vi "ExcelWrite.vi"(6 "Start Position":cluster{"Sheet":i32, "Row":i32, "Column":i32}={"Sheet"=0, "Row"=1, "Column"=2}, 9 "Values":string[][][](array[string]), 10 "Report Name":path, 11 "Module File":path) -> ()   [LabVIEW 2014]
uses:
  Data/Polymorphic VIs/Set Cell (String).vi
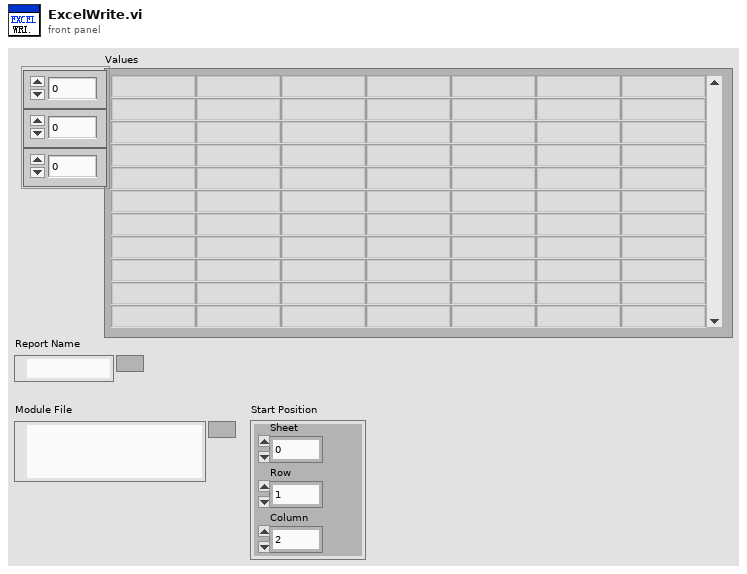
[diagram p1: front panel]
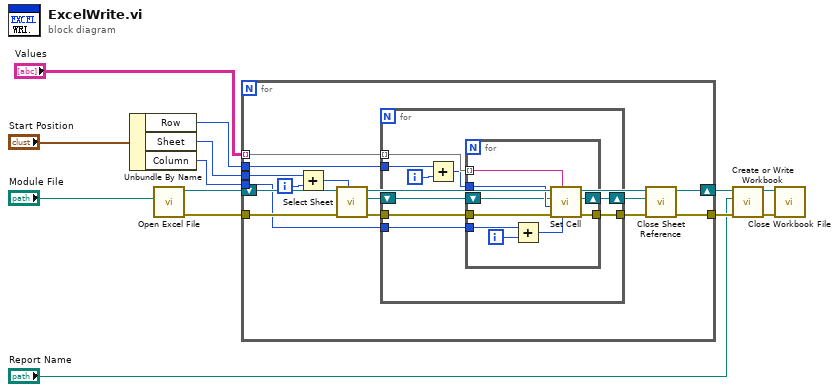
[diagram p0: block diagram]
diagram:
  n1 = Unbundle By Name("Start Position") -> ("Row"=w11:i32, "Sheet"=w5:i32, "Column"=w4:i32)
  n2 = call "Open Excel File.vi"("File Name"="Module File") -> ("error out"=w10:errorcluster, "IWorkbook Reference Out"=w13:refnum<k24>)  [unwired: 9 in]
  n3 = for {
    tunnel: "Values" -> [w21] mode=indexing
    tunnel: w5 -> [w25]
    tunnel: w4 -> [w19]
    tunnel: w11 -> [w20]
    tunnel: w10 -> [w23]
    tunnel: [w15] -> w9
    shift-right: [w22] -> w8
    shift-left: w13 -> [w27]
    i -> [w26]
    n4 = Add(x=w25, y=w26) -> (x+y=w24:i32)
    n5 = call "Select Sheet.vi"("Sheet (0)"=w24, "error in (no error)"=w23, "IWorkbook Reference"=w27) -> ("error out"=w18:errorcluster, "Sheet Reference"=w14:refnum<k24>, "IWorkbook Reference"=w22:refnum<k24>)  [unwired: 6 in]
    n6 = for {
      tunnel: w21 -> [w36] mode=indexing
      tunnel: w20 -> [w34]
      tunnel: w19 -> [w33]
      tunnel: [w31] -> w16
      tunnel: w18 -> [w30]
      shift-right: [w29] -> w17
      shift-left: w14 -> [w28]
      i -> [w35]
      n7 = Add(x=w34, y=w35) -> (x+y=w32:i32)
      n8 = for {
        tunnel: w36 -> [w45] mode=indexing
        tunnel: w33 -> [w43]
        tunnel: w32 -> [w41]
        tunnel: [w39] -> w31
        tunnel: w30 -> [w38]
        shift-right: [w37] -> w29
        shift-left: w28 -> [w40]
        i -> [w44]
        n9 = Add(x=w43, y=w44) -> (x+y=w42:i32)
        n10 = call-poly "Set Cell.vi"("Column"=w42, "Value"=w45, "error in (no error)"=w38, "Row"=w41, "Sheet Reference"=w40) -> ("error out"=w39:errorcluster, "Sheet Reference out"=w37:refnum<k24>)  [unwired: 5 in]
      }
    }
    n11 = call "Close Sheet Reference.vi"("error in (no error)"=w16, "Sheet Reference"=w17) -> ("error out"=w15:errorcluster)  [unwired: 9 in]
  }
  n12 = call "Create or Write Workbook.vi"("error in (no error)"=w9, "File Name"="Report Name", "IWorkbook Reference"=w8) -> ("error out"=w7:errorcluster, "IWorkbook Reference Out"=w6:refnum<k24>)  [unwired: 7 in]
  n13 = call "Close Workbook File.vi"("error in (no error)"=w7, "IWorkbook Reference"=w6) -> ()  [unwired: 9 in, 1 out]
